vi "Maxi Gauge-Get Error Status.vi"(8 "Fehler (Eingang)":errorcluster, 10 "Node address":i8=-1 min=-1 max=31 step=1, 11 "VISA-Ressource in":refnum<visa-resource-name>) -> (0 "Fehler (Ausgang)":errorcluster, 1 "Sensor Errorstatus":u16, 2 "MG Errorstatus":u16, 3 "VISA-Ressource out":refnum<visa-resource-name>, 4 "Errortext":string[](array[string]))   [LabVIEW 2012, in "Maxi Gauge.lvlib"]
uses:
  Maxi Gauge.lvlib
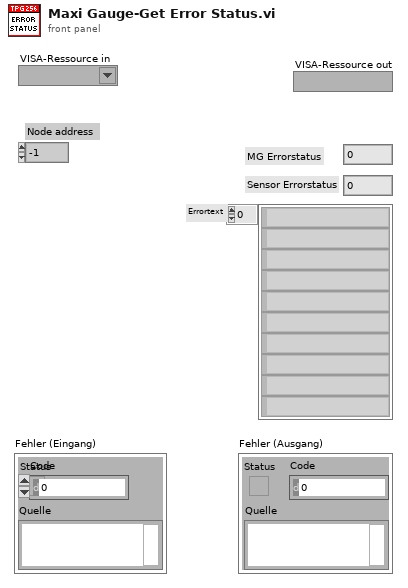
[diagram p1: front panel]
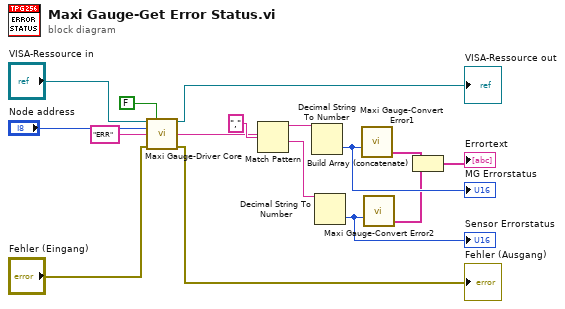
[diagram p0: block diagram]
diagram:
  n1 = call "Maxi Gauge-Driver Core.vi"("VISA-Ressource in"="VISA-Ressource in", "Write/Read"=FALSE, "Node address"="Node address", "Command"="ERR", "Fehler (Eingang)"="Fehler (Eingang)") -> ("VISA-Ressource out"=→"VISA-Ressource out":refnum<visa-resource-name>, "String Out"=w6:string, "Fehler (Ausgang)"=→"Fehler (Ausgang)":errorcluster)  [unwired: 8 in]
  n2 = Match Pattern(string=w6, regular expression=",") -> (before substring=w10:string, after substring=w9:string)  [unwired: 1 in, 2 out]
  n3 = Decimal String To Number(string=w10) -> (number=w15:i32)  [unwired: 2 in, 1 out]
  "MG Errorstatus" <- w15
  n4 = Decimal String To Number(string=w9) -> (number=w13:i32)  [unwired: 2 in, 1 out]
  "Sensor Errorstatus" <- w13
  n5 = call "Maxi Gauge-Convert Error1.vi"("Errorwort1"=w15) -> ("Error Text"=w8:string[])  [unwired: 4 in]
  n6 = call "Maxi Gauge-Convert Error2.vi"("Errorwort1"=w13) -> ("Error Text"=w7:string[])  [unwired: 4 in]
  n7 = Build Array (concatenate)(w8, w7) -> (→"Errortext":string[])
